vi "PH_VacuumControl.set i Attr and open Services.vi"(0 "i ref in":refnum<vi>, 5 "error in (no error)":errorcluster) -> (14 "i ref out":refnum<vi>, 16 "i Attributes":T1={"GUI Refs"={"Exit"=refnum, "Set Unit"=refnum, "Device found"=refnum, "Busy"=refnum, "State"=refnum, "Delete"=refnum, "Channels"=refnum, "Channel Name"=refnum, "Trend"=refnum, "Logarithmic"=refnum, "Limit reached"=refnum, "Channel Name 1 MT"=refnum, "Channel Name 2 MT"=refnum, "Trend MT"=refnum, "Logarithmic MT"=refnum, "Limit reached MT"=refnum}, "Device found"=FALSE, "Busy"=FALSE, "Selected Unit"=1, "Channels [mbar]"={"Channel 1"=99999.0, "Channel 2"=99999.0, "Channel 3"=99999.0, "Channel 4"=99999.0, "Channel 5"=99999.0, "Channel 6"=99999.0, "Name Channel 1"="", "Name Channel 2"="", "Name Channel 3"="", "Name Channel 4"="", "Name Channel 5"="", "Name Channel 6"="", "Upper Limit"=0.0, "Upper Limit 2"=0.0, "Upper Limit 3"=0.0, "Upper Limit 4"=0.0, "Upper Limit 5"=0.0, "Upper Limit 6"=0.0}, "Channel Names"={"Channel 1"="N/A", "Channel 2"="N/A", "Channel 3"="N/A", "Channel 4"="N/A", "Channel 5"="N/A", "Channel 6"="N/A"}, "Status"=0, "AGCxxx VISA Cluster"={"VISA resource name"="", "VISA Timeout Value (1000 ms)"=1000, "Lock Timeout (1000 ms)"=1000, "MAX Channel (6)"=6}, "Instr Firmware Revision"="N/A", "Service IDs Pressure"={"Channel 1"=-1, "Channel 2"=-1, "Channel 3"=-1, "Channel 4"=-1, "Channel 5"=-1, "Channel 6"=-1}, "Service IDs Limits"={"Channel 1"=-1, "Channel 2"=-1, "Channel 3"=-1, "Channel 4"=-1, "Channel 5"=-1, "Channel 6"=-1}, "Trend"={"Start Point"=timestamp(0 s since 1904-01-01), "Pressures [mbar] Channel 1"=[], "Pressures [mbar] Channel 2"=[], "Pressures [mbar] Channel 3"=[], "Pressures [mbar] Channel 4"=[], "Pressures [mbar] Channel 5"=[], "Pressures [mbar] Channel 6"=[], "Timebase [s]"=[], "Trend Channel"=0, "Start Fit"=0.0, "Trend Channel 1 MT"=0, "Trend Channel 2 MT"=0, "Start or continue Fit MT"=0.0, "Continue or start Fit MT"=0.0, "Datasets strored"=0, "Dataarray Size"=0}, "Running"=FALSE} {"Status" items=["no info", "off/false/out", "on/true/in", "Failure", "Alarm", "Status 1", "Status 2", "Status 3"]; "Channels [mbar]"."Upper Limit 6" format="%.4e"; "Channels [mbar]"."Upper Limit 5" format="%.4e"; "Channels [mbar]"."Upper Limit 4" format="%.4e"; "Channels [mbar]"."Upper Limit 3" format="%.4e"; "Channels [mbar]"."Upper Limit 2" format="%.4e"; "Channels [mbar]"."Upper Limit" format="%.4e"; "Channels [mbar]"."Channel 6" format="%.4e"; "Channels [mbar]"."Channel 5" format="%.4e"; "Channels [mbar]"."Channel 4" format="%.4e"; "Channels [mbar]"."Channel 3" format="%.4e"; "Channels [mbar]"."Channel 2" format="%.4e"; "Channels [mbar]"."Channel 1" format="%.4e"; "Selected Unit" items=["mBar", "Pascal", "Torr"]}, 19 "error out":errorcluster)   [LabVIEW 2014, in "PH_VacuumControl.lvlib"]
doc: "This VI sets own Attributes and starts DIM services."
uses:
  PH_VacuumControl.lvlib
  PH_VacuumControl.i attribute.ctl
  PH_VacuumControl.Channels.ctl
  PH_Basics/PH_StatusHandler/PH_StatusHandler.Status.ctl
  instr.lib/AGCxxx/AGCxxx/AGCxxx VISA Control.ctl
  PH_Basics/PH_Common/PH_Common.lvlib
  instr.lib/AGCxxx/AGCxxx - Driver.lvlib
  CS_Core/CSSystem/CSSystemLib/CSSystemLib.lvlib
  PH_Basics/PH_StatusHandler/PH_StatusHandler.lvlib
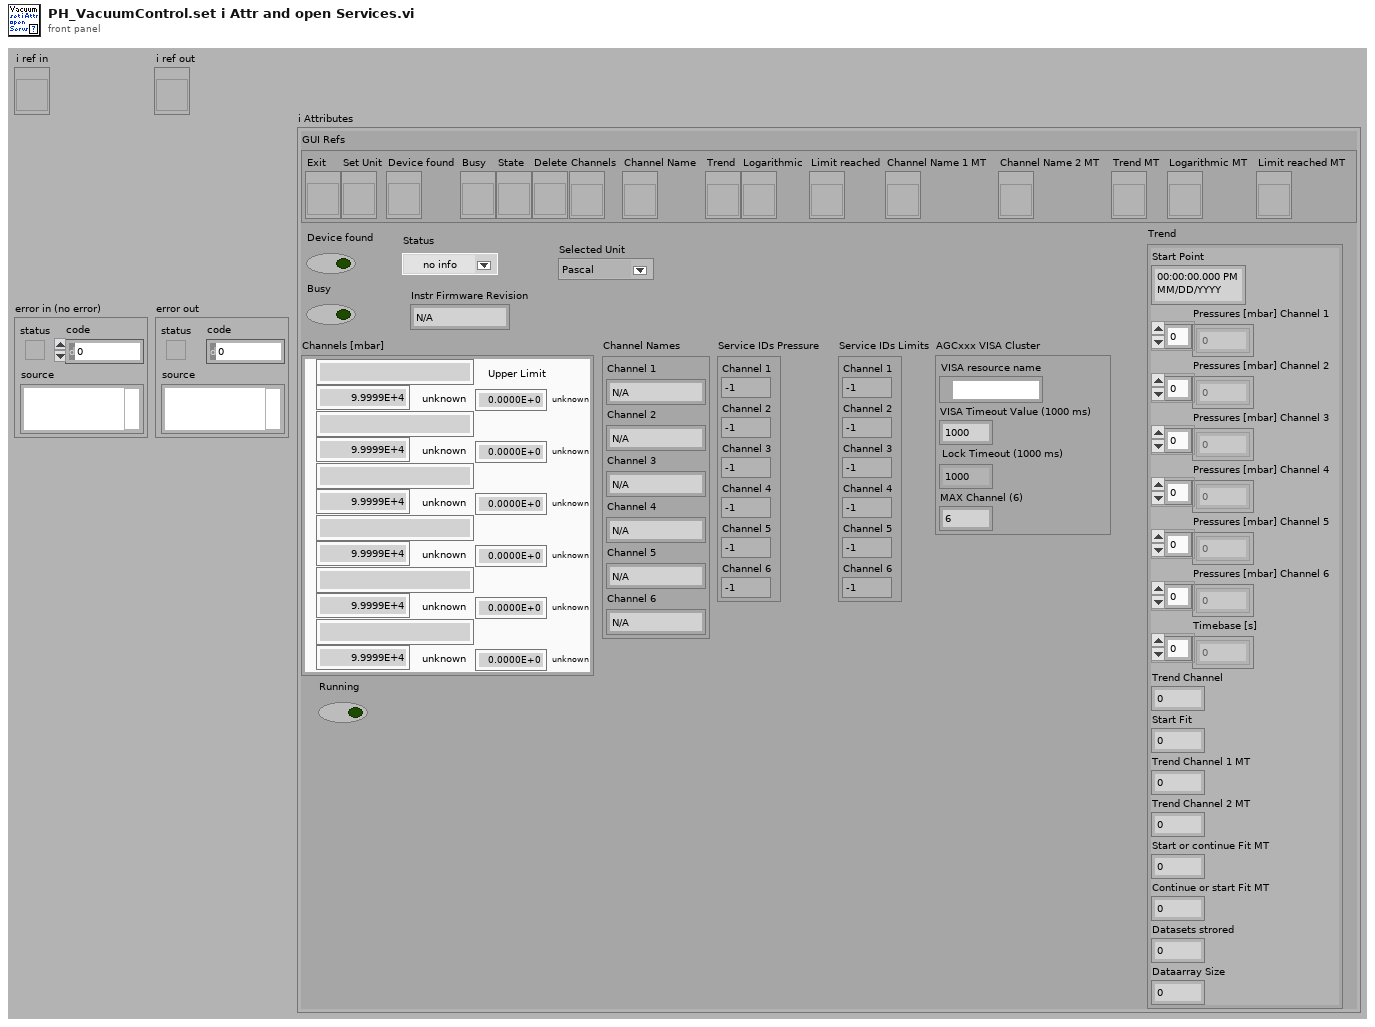
[diagram p1: front panel]
types:
  T1 = typedef "PH_VacuumControl.lvlib/PH_VacuumControl.i attribute.ctl" = cluster{"GUI Refs":cluster{"Exit":refnum<vi>, "Set Unit":refnum<vi>, "Device found":refnum<vi>, "Busy":refnum<vi>, "State":refnum<vi>, "Delete":refnum<vi>, "Channels":refnum<vi>, "Channel Name":refnum<vi>, "Trend":refnum<vi>, "Logarithmic":refnum<vi>, "Limit reached":refnum<vi>, "Channel Name 1 MT":refnum<vi>, "Channel Name 2 MT":refnum<vi>, "Trend MT":refnum<vi>, "Logarithmic MT":refnum<vi>, "Limit reached MT":refnum<vi>}, "Device found":bool, "Busy":bool, "Selected Unit":i32, "Channels [mbar]":T2, "Channel Names":cluster{"Channel 1":string, "Channel 2":string, "Channel 3":string, "Channel 4":string, "Channel 5":string, "Channel 6":string}, "Status":T3, "AGCxxx VISA Cluster":T4, "Instr Firmware Revision":string, "Service IDs Pressure":cluster{"Channel 1":i32, "Channel 2":i32, "Channel 3":i32, "Channel 4":i32, "Channel 5":i32, "Channel 6":i32}, "Service IDs Limits":cluster{"Channel 1":i32, "Channel 2":i32, "Channel 3":i32, "Channel 4":i32, "Channel 5":i32, "Channel 6":i32}, "Trend":cluster{"Start Point":timestamp, "Pressures [mbar] Channel 1":dbl[], "Pressures [mbar] Channel 2":dbl[], "Pressures [mbar] Channel 3":dbl[], "Pressures [mbar] Channel 4":dbl[], "Pressures [mbar] Channel 5":dbl[], "Pressures [mbar] Channel 6":dbl[], "Timebase [s]":i32[], "Trend Channel":u16, "Start Fit":dbl, "Trend Channel 1 MT":u16, "Trend Channel 2 MT":u16, "Start or continue Fit MT":dbl, "Continue or start Fit MT":dbl, "Datasets strored":i32, "Dataarray Size":i32}, "Running":bool}
  T2 = typedef "PH_VacuumControl.lvlib/PH_VacuumControl.Channels.ctl" = cluster{"Channel 1":dbl, "Channel 2":dbl, "Channel 3":dbl, "Channel 4":dbl, "Channel 5":dbl, "Channel 6":dbl, "Name Channel 1":string, "Name Channel 2":string, "Name Channel 3":string, "Name Channel 4":string, "Name Channel 5":string, "Name Channel 6":string, "Upper Limit":dbl, "Upper Limit 2":dbl, "Upper Limit 3":dbl, "Upper Limit 4":dbl, "Upper Limit 5":dbl, "Upper Limit 6":dbl}
  T3 = typedef "PH_StatusHandler.lvlib/PH_StatusHandler.Status.ctl" = i16
  T4 = typedef "AGCxxx - Driver.lvlib/AGCxxx VISA Control.ctl" = cluster{"VISA resource name":refnum<visa-resource-name>, "VISA Timeout Value (1000 ms)":u32, "Lock Timeout (1000 ms)":u32, "MAX Channel (6)":i32}
  T5 = cluster{"[0]":i32, "[1]":i32, "[2]":i32, "[3]":i32, "[4]":i32, "[5]":i32}
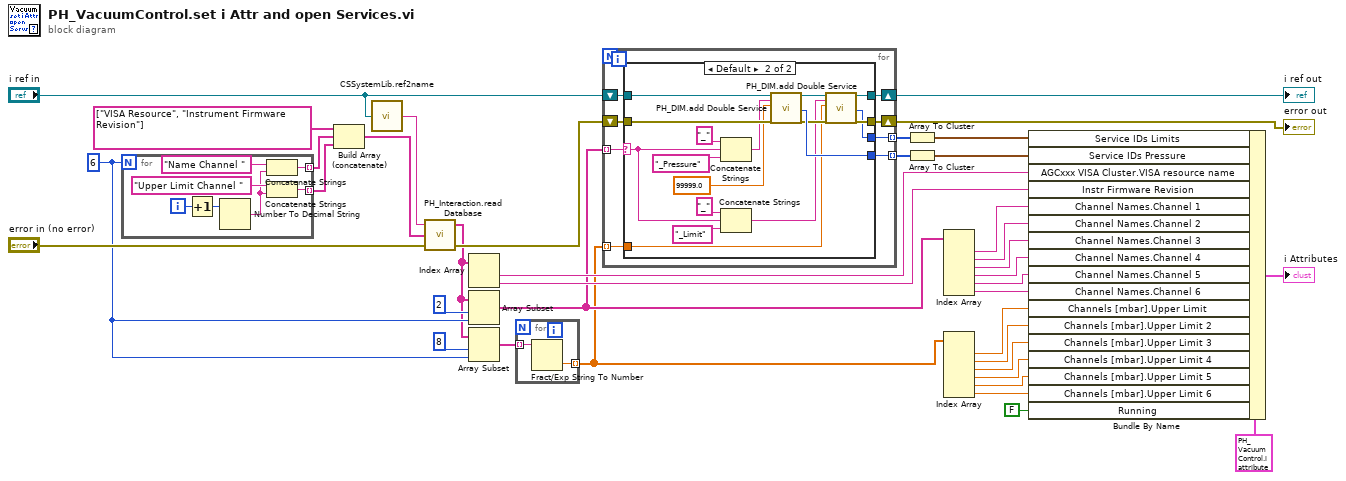
[diagram p0: block diagram]
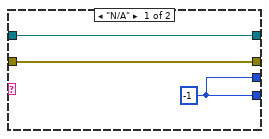
[diagram p2: hidden frame]
diagram:
  w4 = 6
  n1 = for {
    N: w4 -> [_]
    tunnel: [w40] -> w8 mode=indexing
    tunnel: [w39] -> w9 mode=indexing
    i -> [w45]
    n2 = Increment(x=w45) -> (x+1=w44:i32)
    n3 = Number To Decimal String(number=w44) -> (decimal integer string=w41:string)  [unwired: 1 in]
    n4 = Concatenate Strings("Name Channel " ("string"), w41) -> (w39:string)
    n5 = Concatenate Strings("Upper Limit Channel " ("string"), w41) -> (w40:string)
  }
  n6 = Build Array (concatenate)(string[] ["VISA Resource", "Instrument Firmware Revision"] ("Strings to search for"), w9, w8) -> (w10:string[])
  n7 = call "CSSystemLib.ref2name.vi"("obj refnum"="i ref in") -> ("name"=w14:string)
  n8 = call "PH_Interaction.read Database.vi"("error in (no error)"="error in (no error)", "Strings to search for"=w10, "DB Entry to read"=w14) -> ("error out"=w16:errorcluster, "Values"=w2:string[])  [unwired: 1 in]
  n9 = Index Array(array=w2) -> (element #1=w13:string, element #2=w12:string)  [unwired: 2 in]
  n10 = Array Subset(array=w2, index=2, length=w4) -> (w6:string[])
  n11 = Array Subset(array=w2, index=8, length=w4) -> (w3:string[])
  n12 = for {
    tunnel: w3 -> [w47] mode=indexing
    tunnel: [w46] -> w1 mode=indexing
    n13 = Fract/Exp String To Number(string=w47) -> (number=w46:dbl)  [unwired: 3 in, 1 out]
  }
  n14 = for {
    shift-right: [w55] -> w20
    shift-left: w16 -> [w54]
    tunnel: w6 -> [w53] mode=indexing
    shift-right: [w51] -> w21
    shift-left: "i ref in" -> [w52]
    tunnel: [w50] -> w24 mode=indexing
    tunnel: w1 -> [w49] mode=indexing
    tunnel: [w48] -> w23 mode=indexing
    n15 = case shown="Default" w53 {
      selector: w53 -> [_ w66]
      tunnel: [w58 w62] -> w55
      tunnel: w54 -> [w58 w74]
      tunnel: w52 -> [w57 w75]
      tunnel: [w57 w64] -> w51
      tunnel: [w56 w69] -> w50
      tunnel: w49 -> [_ w60]
      tunnel: [w56 w59] -> w48
      frame "N/A" {
        w56 = -1 ("Service ID")
      }
      frame Default {
        n16 = Concatenate Strings("_" ("string"), w66, "_Pressure" ("string")) -> (w71:string)
        n17 = Concatenate Strings("_" ("string"), w66, "_Limit" ("string")) -> (w61:string)
        n18 = call "PH_DIM.add Double Service.vi"("i ref in"=w75, "Service Name"=w71, "Double Value"=99999.0 ("Number"), "error in (no error)"=w74) -> ("i ref out"=w65:refnum<vi>, "Service ID"=w69:i32, "error out"=w63:errorcluster)  [unwired: 13 in]
        n19 = call "PH_DIM.add Double Service.vi"("i ref in"=w65, "Service Name"=w61, "Double Value"=w60, "error in (no error)"=w63) -> ("i ref out"=w64:refnum<vi>, "Service ID"=w59:i32, "error out"=w62:errorcluster)  [unwired: 13 in]
      }
    }
  }
  "error out" <- w20
  "i ref out" <- w21
  n20 = Array To Cluster(array=w23) -> (cluster=w19:T5)
  n21 = Array To Cluster(array=w24) -> (cluster=w22:T5)
  n22 = Index Array(array=w6) -> (element #1=w38:string, element #2=w37:string, element #3=w36:string, element #4=w35:string, element #5=w34:string, element #6=w33:string)  [unwired: 6 in]
  n23 = Index Array(array=w1) -> (element #1=w31:dbl, element #2=w32:dbl, element #3=w30:dbl, element #4=w29:dbl, element #5=w28:dbl, element #6=w27:dbl)  [unwired: 6 in]
  n24 = Bundle By Name(cluster=T1 {"GUI Refs"={"Exit"=refnum, "Set Unit"=refnum, "Device found"=refnum, "Busy"=refnum, "State"=refnum, "Delete"=refnum, "Channels"=refnum, "Channel Name"=refnum, "Trend"=refnum, "Logarithmic"=refnum, "Limit reached"=refnum, "Channel Name 1 MT"=refnum, "Channel Name 2 MT"=refnum, "Trend MT"=refnum, "Logarithmic MT"=refnum, "Limit reached MT"=refnum}, "Device found"=FALSE, "Busy"=FALSE, "Selected Unit"=1, "Channels [mbar]"={"Channel 1"=99999.0, "Channel 2"=99999.0, "Channel 3"=99999.0, "Channel 4"=99999.0, "Channel 5"=99999.0, "Channel 6"=99999.0, "Name Channel 1"="", "Name Channel 2"="", "Name Channel 3"="", "Name Channel 4"="", "Name Channel 5"="", "Name Channel 6"="", "Upper Limit"=0.0, "Upper Limit 2"=0.0, "Upper Limit 3"=0.0, "Upper Limit 4"=0.0, "Upper Limit 5"=0.0, "Upper Limit 6"=0.0}, "Channel Names"={"Channel 1"="N/A", "Channel 2"="N/A", "Channel 3"="N/A", "Channel 4"="N/A", "Channel 5"="N/A", "Channel 6"="N/A"}, "Status"=0, "AGCxxx VISA Cluster"={"VISA resource name"="", "VISA Timeout Value (1000 ms)"=1000, "Lock Timeout (1000 ms)"=1000, "MAX Channel (6)"=6}, "Instr Firmware Revision"="N/A", "Service IDs Pressure"={"Channel 1"=-1, "Channel 2"=-1, "Channel 3"=-1, "Channel 4"=-1, "Channel 5"=-1, "Channel 6"=-1}, "Service IDs Limits"={"Channel 1"=-1, "Channel 2"=-1, "Channel 3"=-1, "Channel 4"=-1, "Channel 5"=-1, "Channel 6"=-1}, "Trend"={"Start Point"=timestamp(0 s since 1904-01-01), "Pressures [mbar] Channel 1"=[], "Pressures [mbar] Channel 2"=[], "Pressures [mbar] Channel 3"=[], "Pressures [mbar] Channel 4"=[], "Pressures [mbar] Channel 5"=[], "Pressures [mbar] Channel 6"=[], "Timebase [s]"=[], "Trend Channel"=0, "Start Fit"=0.0, "Trend Channel 1 MT"=0, "Trend Channel 2 MT"=0, "Start or continue Fit MT"=0.0, "Continue or start Fit MT"=0.0, "Datasets strored"=0, "Dataarray Size"=0}, "Running"=FALSE} ("i attribute"), "Service IDs Limits"=w19, "Service IDs Pressure"=w22, "AGCxxx VISA Cluster.VISA resource name"=w13, "Instr Firmware Revision"=w12, "Channel Names.Channel 1"=w38, "Channel Names.Channel 2"=w37, "Channel Names.Channel 3"=w36, "Channel Names.Channel 4"=w35, "Channel Names.Channel 5"=w34, "Channel Names.Channel 6"=w33, "Channels [mbar].Upper Limit"=w31, "Channels [mbar].Upper Limit 2"=w32, "Channels [mbar].Upper Limit 3"=w30, "Channels [mbar].Upper Limit 4"=w29, "Channels [mbar].Upper Limit 5"=w28, "Channels [mbar].Upper Limit 6"=w27, "Running"=FALSE) -> (→"i Attributes":T1)
